vi "FuelPump.vi"(11 "Fuel Loading":bool) -> (0 "Solenoids":bool[](array[boolean]), 3 "Fuel Pump":bool)   [LabVIEW 2016]
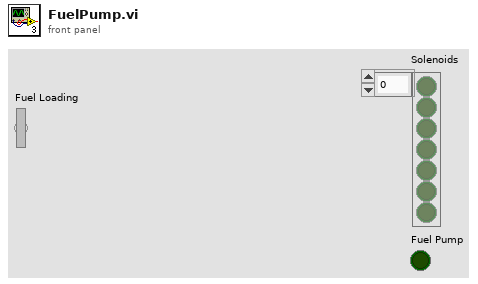
[diagram p1: front panel]
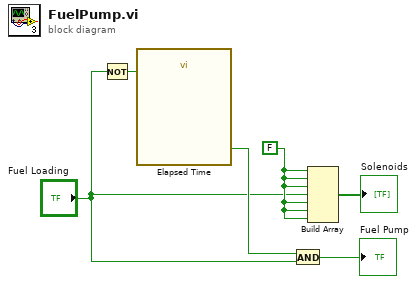
[diagram p0: block diagram]
diagram:
  w6 = FALSE
  n1 = Not(x="Fuel Loading") -> (.not. x?=w2:bool)
  n2 = call "Elapsed Time"("Reset"=w2) -> ("Time has Elapsed"=w3:bool)  [unwired: 11 in, 7 out]
  n3 = And(x=w3, y="Fuel Loading") -> (x .and. y?=→"Fuel Pump":bool)
  n4 = Build Array(w6, w6, w6, "Fuel Loading", w6, w6, w6) -> (→"Solenoids":bool[])
